vi "TX-BPCS-SIM-UDP (SubVI).vi"(7 "BPCS-SIM-TX-ARRAY in":dbl[](array[numeric]), 8 "error in (no error)":errorcluster, 9 "UDP Network Connection in":refnum<k16>, 10 "SIM-PC-IP":u32, 11 "SIM-PC-UDP-Port":u16) -> (0 "error out":errorcluster, 1 "length":i32[](array[numeric]), 2 "BPCS-SIM-TX-ARRAY out":dbl[](array[numeric]), 3 "UDP Network Connection out":refnum<k16>)   [LabVIEW 2018]
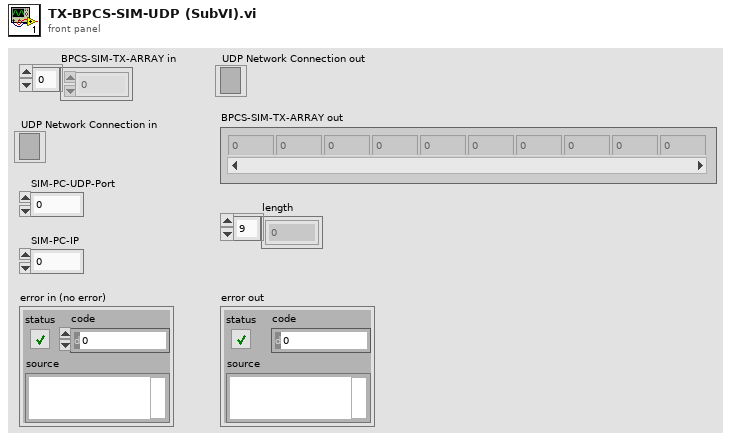
[diagram p1: front panel]
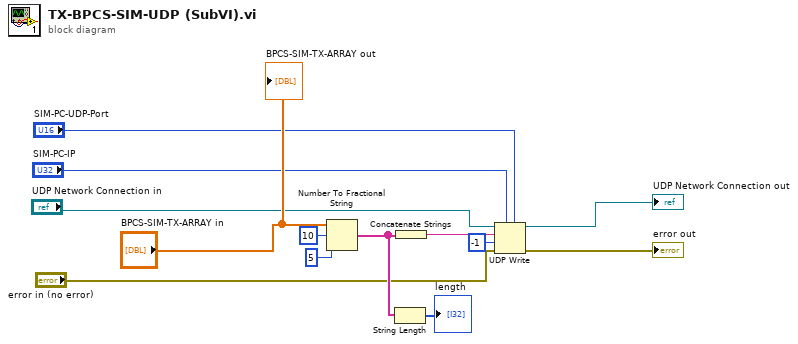
[diagram p0: block diagram]
diagram:
  n1 = Number To Fractional String(number="BPCS-SIM-TX-ARRAY in", width (-)=i16 10, precision (6)=i16 5) -> (F-format string=w8:string[])  [unwired: 1 in]
  n2 = String Length(string=w8) -> (length=→"length":i32[])
  n3 = Concatenate Strings(w8) -> (w1:string)
  n4 = UDP Write(address="SIM-PC-IP", port or service name="SIM-PC-UDP-Port", connection ID="UDP Network Connection in", data in=w1, 8:"error in (no error)", 9:-1 ("timeout ms (25000)")) -> (error out=→"error out":errorcluster, 3:→"UDP Network Connection out":refnum<k16>)
  "BPCS-SIM-TX-ARRAY out" <- "BPCS-SIM-TX-ARRAY in"
